vi "ingest.video-with_manifest_timestamp.vi"(6 "Properties and Labels":cluster{"Properties":string, "Labels":string}, 7 "Timestamp S3 Path":string, 8 "error in":errorcluster, 9 "Title and Description":cluster{"Title":string, "Description":string}, 10 "S3 Path":string, 11 "Nominal Client in":refnum<class "Nominal Client.lvclass">) -> (0 "error out":errorcluster, 1 "Response":T1, 2 "Video RID":string, 3 "Nominal Client out":refnum<class "Nominal Client.lvclass">, 4 "Response":string)   [LabVIEW 2020, in "Nominal Client.lvclass"]
doc: "Ingests video data from a S3 Nominal upload bucket."
uses:
  Nominal Client.lvclass
  4b965f09-dc68-4d5e-a5c1-32d476accfd4.vi
  <vilib>/JDP Science/JSONtext/JSON text to Variant.vi
  <vilib>/JDP Science/JSONtext/LVClass Serializer/JSONtext LVClass Serializer.lvclass
  Nominal Client.lvclass/Nominal Client.ctl
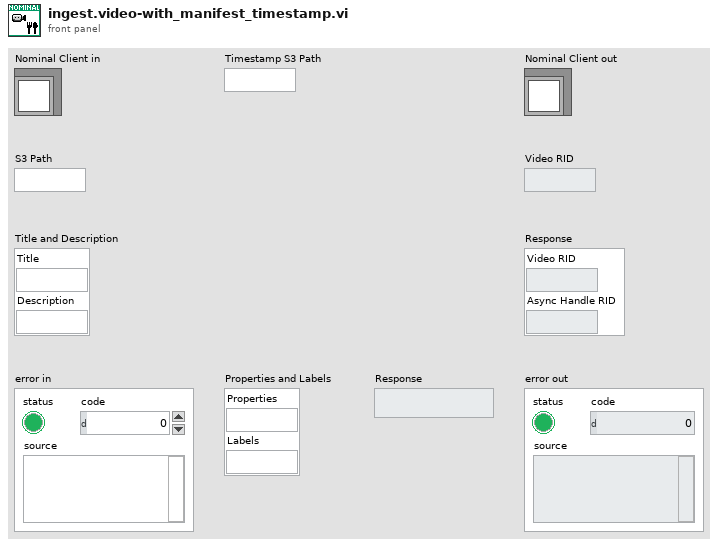
[diagram p1: front panel]
types:
  T1 = cluster{"Video RID":string, "Async Handle RID":string}
  T2 = cluster{"Timestamp Manifests":cluster{"type":string, "timestampManifests":cluster{"sources":cluster{"type":string, "s3":cluster{"path":string}}}}}
  T3 = cluster{"videoRid":string, "asyncHandle":cluster{"rid":string}}
  T4 = cluster{"type":string, "s3":cluster{"path":string}}
  T5 = cluster{"source":cluster{"type":string, "s3":cluster{"path":string}}, "properties":string, "labels":string, "timestamps":cluster{"Timestamp Manifests":cluster{"type":string, "timestampManifests":cluster{"sources":cluster{"type":string, "s3":cluster{"path":string}}}}}, "title":string, "description":string}
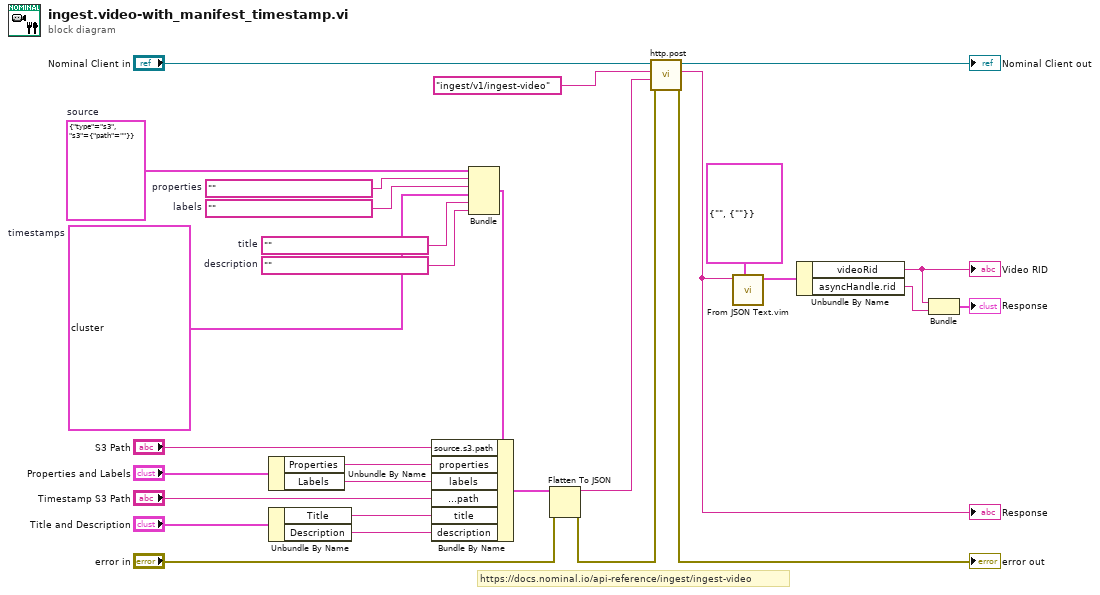
[diagram p0: block diagram]
diagram:
  w11 = ""  # description
  w12 = ""  # title
  w13 = T2 {"Timestamp Manifests"={"type"="timestampManifests", "timestampManifests"={"sources"={"type"="s3", "s3"={"path"=""}}}}}  # timestamps
  w14 = ""  # labels
  w15 = ""  # properties
  w25 = T4 {"type"="s3", "s3"={"path"=""}}  # source
  # "https://docs.nominal.io/api-reference/ingest/ingest-video"
  n1 = Unbundle By Name("Properties and Labels") -> ("Properties"=w7:string, "Labels"=w6:string)
  n2 = Unbundle By Name("Title and Description") -> ("Title"=w4:string, "Description"=w3:string)
  n3 = Bundle("source"=w25, "properties"=w15, "labels"=w14, "timestamps"=w13, "title"=w12, "description"=w11) -> (w10:T5)  [unwired: 1 in]
  n4 = Bundle By Name(cluster=w10, "source.s3.path"="S3 Path", "properties"=w7, "labels"=w6, "timestamps.Timestamp Manifests.timestampManifests.sources.s3.path"="Timestamp S3 Path", "title"=w4, "description"=w3) -> (w2:T5)
  n5 = Flatten To JSON(anything=w2, error in (no error)="error in") -> (JSON string=w24:string, 11:w23:errorcluster)  [unwired: 1 in]
  n6 = call "http.post.vi"("error in"=w23, "Request body"=w24, "Path"="ingest/v1/ingest-video", "Nominal Client in"="Nominal Client in") -> ("error out"=→"error out":errorcluster, "Response"=w20:string, "Nominal Client out"=→"Nominal Client out":refnum<class "Nominal Client.lvclass">)  [unwired: 4 in, 1 out]
  "Response" <- w20
  n7 = call "From JSON Text.vim"("Data Type and Default Value"=T3 {"videoRid"="", "asyncHandle"={"rid"=""}} ("Information"), "JSON"=w20) -> ("Data out"=w19:T3)  [unwired: 8 in, 1 out]
  n8 = Unbundle By Name(w19) -> ("videoRid"=w18:string, "asyncHandle.rid"=w17:string)
  "Video RID" <- w18
  n9 = Bundle("videoRid"=w18, "rid"=w17) -> (→"Response":cluster{"videoRid":string, "rid":string})  [unwired: 1 in]
